vi "Create HDF5 chunked dataset (2D).vi"(5 "block size":u32, 6 "compression":u8, 7 "number of channels":i32, 8 "error in (no error)":errorcluster, 9 "data type":variant, 10 "name":string="stuff", 11 "ref in":T1 format="%.0x") -> (0 "error out":errorcluster, 3 "dset out":i32)   [LabVIEW 2012, in "h5logger.lvlib"]
uses:
  h5logger.lvlib
  <vilib>/addons/h5labview2/dataset/H5D.lvlib
  <vilib>/addons/h5labview2/space/H5S.lvlib
  <vilib>/addons/h5labview2/props/H5P.lvlib
  <vilib>/addons/h5labview2/type/H5T.lvlib
  <vilib>/addons/h5labview2/base/hid_t.ctl
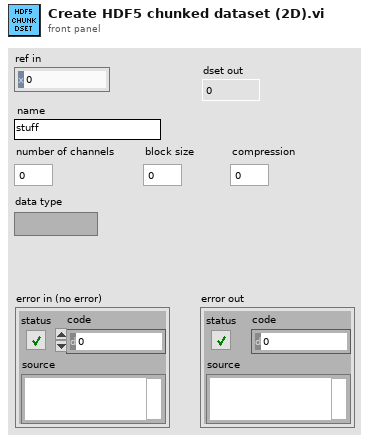
[diagram p1: front panel]
types:
  T1 = typedef "hid_t.ctl" = i32
  T2 = enum16{"H5P_ROOT", "H5P_OBJECT_CREATE", "H5P_FILE_CREATE", "H5P_FILE_ACCESS", "H5P_DATASET_CREATE", "H5P_DATASET_ACCESS", "H5P_DATASET_XFER", "H5P_FILE_MOUNT", "H5P_GROUP_CREATE", "H5P_GROUP_ACCESS", "H5P_DATATYPE_CREATE", "H5P_DATATYPE_ACCESS", "H5P_STRING_CREATE", "H5P_ATTRIBUTE_CREATE", "H5P_OBJECT_COPY", "H5P_LINK_CREATE", "H5P_LINK_ACCESS"}
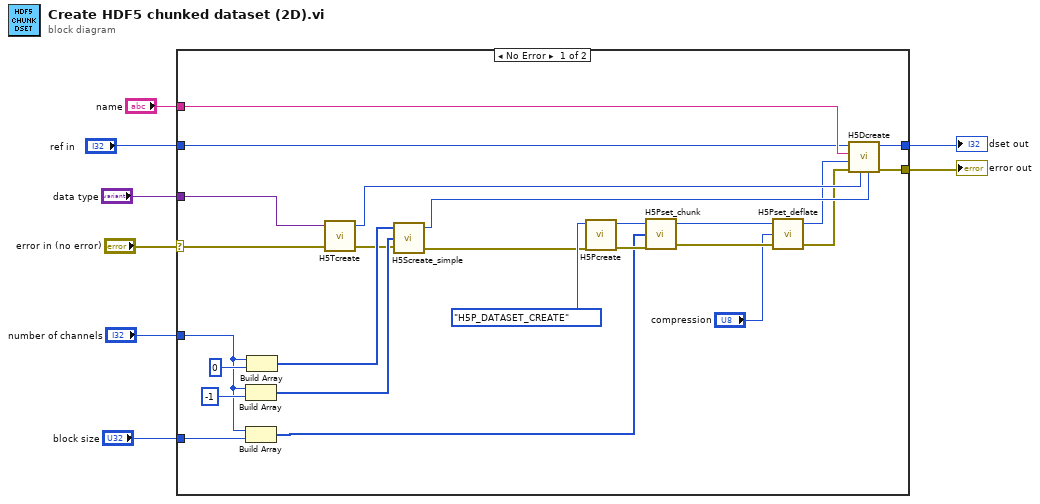
[diagram p0: block diagram]
diagram:
  n1 = case shown="No Error" "error in (no error)" {
    selector: "error in (no error)" -> [w10 w34]
    tunnel: [w33 w34] -> w8
    tunnel: [w32 _] -> w7
    tunnel: "name" -> [w26 _]
    tunnel: "ref in" -> [w25 _]
    tunnel: "data type" -> [w24 _]
    tunnel: "number of channels" -> [w21 _]
    tunnel: "block size" -> [w20 _]
    frame No Error {
      n2 = Build Array(w21, -1 ("element")) -> (w19:i32[])
      n3 = Build Array(w21, w20) -> (w17:u32[])
      n4 = Build Array(w21, 0 ("element")) -> (w18:i32[])
      n5 = call <vilib>:"H5Tcreate.vi"("error in (no error)"=w10, "type variant"=w24) -> ("error out"=w16:errorcluster, "type out"=w30:i32)  [unwired: 2 in]
      n6 = call <vilib>:"H5Screate_simple.vi"("error in (no error)"=w16, "maxdims"=w19, "dims"=w18) -> ("error out"=w15:errorcluster, "space out"=w31:T1)  [unwired: 1 out]
      n7 = call <vilib>:"H5Pcreate.vi"("error in (no error)"=w15, "prop class (DATASET_CREATE)"=T2."H5P_DATASET_CREATE" ("prop class")) -> ("error out"=w28:errorcluster, "ref out"=w29:T1)  [unwired: 4 in]
      n8 = call <vilib>:"H5Pset_chunk.vi"("error in (no error)"=w28, "chunk size"=w17, "prop in"=w29) -> ("error out"=w13:errorcluster, "prop out"=w14:T1)  [unwired: 1 in]
      n9 = call <vilib>:"H5Pset_deflate.vi"("error in (no error)"=w13, "level"="compression", "prop in"=w14) -> ("error out"=w11:errorcluster, "prop out"=w12:T1)  [unwired: 1 in]
      n10 = call <vilib>:"H5Dcreate.vi"("space id"=w31, "type id"=w30, "error in (no error)"=w11, "props id"=w12, "name"=w26, "loc in"=w25) -> ("error out"=w33:errorcluster, "dset out"=w32:T1)  [unwired: 2 in]
    }
    frame Error {
    }
  }
  "error out" <- w8
  "dset out" <- w7
